vi "Initialize lock in.vi"(6 "Internal Reference Frequency (1000 Hz)":dbl=1000.0, 7 "Sine Output Amplitude (1 V)":dbl=1.0, 9 "Data Collection":T2={"Sample Rate (0: 62.5 mHz)"=0, "Continuous Storage (T: Enable)"=TRUE, "Number of Points (100)"=100, "Channel (1: Channel 1 Display)"=1, "Channel 1 Display (0: X)"=0} {"Channel 1 Display (0: X)" items=["X", "R", "X Noise", "Aux In 1", "Aux In 2"]; "Channel (1: Channel 1 Display)" items=["Channel 1 Display"=1, "Channel 2 Display"=2]; "Sample Rate (0: 62.5 mHz)" items=["62.5 mHz", "125 mHz", "250 mHz", "500 mHz", "1 Hz", "2 Hz", "4 Hz", "8Hz", "16 Hz", "32 Hz", "64 Hz", "128 Hz", "256 Hz", "512 Hz", "Trigger "]}, 11 "Configure":T3={"Lock in Amplifier PORT"="", "Input Connection (0: Single-Ended Voltage) "=0, "Input Coupling (0: AC)"=0, "Input Notch Filter (0: None)"=0, "Reference Source (1: Internal)"=1, "Dynamic Reserve (-1: Auto Reserve)"=-1, "Sensitivity (-1: Auto gain)"=-1, "Time Constant (8: 100ms)"=8} {"Time Constant (8: 100ms)" items=["10 us", "30 us", "100 us", "300 us", "1 ms", "3 ms", "10 ms", "30 ms", "100 ms", "300 ms", "1 s", "3 s", "10 s", "30 s", "100 s", "300 s", "1 ks", "3 ks", "10 ks", "30 ks"]; "Sensitivity (-1: Auto gain)" items=["Auto Gain"=-1, "2 nV/fA"=0, "5 nV/fA"=1, "10 nV/fA"=2, "20 nV/fA"=3, "50 nV/fA"=4, "100 nV/fA"=5, "200 nV/fA"=6, "500 nV/fA"=7, "1 uV/pA"=8, "2 uV/pA"=9, "5 uV/pA"=10, "10 uV/pA"=11, "20 uV/pA"=12, "50 uV/pA"=13, "100 uV/pA"=14, "200 uV/pA"=15, "500 uV/pA"=16, "1 mV/nA"=17, "2 mV/nA"=18, "5 mV/nA"=19, "10 mV/nA"=20, "20 mV/nA"=21, "50 mV/nA"=22, "100 mV/nA"=23, "200 mV/nA"=24, "500 mV/mA"=25, "1 V/uA"=26]; "Dynamic Reserve (-1: Auto Reserve)" items=["Auto Reserve"=-1, "High Reserve"=0, "Normal"=1, "Low Noise"=2]; "Reference Source (1: Internal)" items=["External", "Internal"]; "Input Notch Filter (0: None)" items=["None", "Line Notch", "2x Line Notch", "Both Notch Filters"]; "Input Coupling (0: AC)" items=["AC", "DC"]; "Input Connection (0: Single-Ended Voltage)" items=["Single-Ended Voltage", "Differential Voltage", "1 MOhm Current Gain", "100 MOhm Current Gain"]}) -> (1 "Output":T1)   [LabVIEW 2020]
uses:
  Downloads/stanford_research_830/Stanford Research 830/Stanford Research 830.lvlib
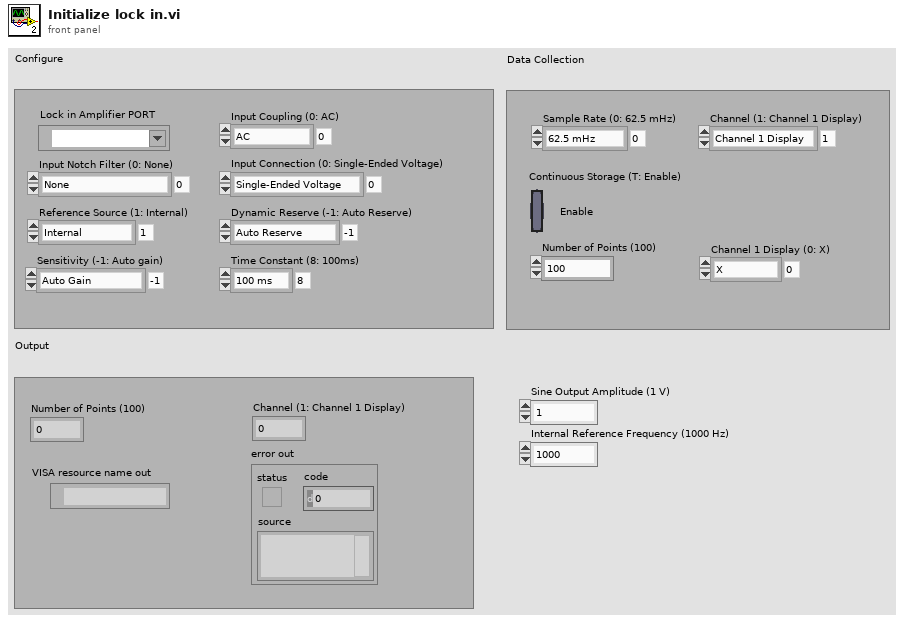
[diagram p1: front panel]
types:
  T1 = cluster{"Number of Points (100)":u32, "VISA resource name out":refnum<visa-resource-name>, "Channel (1: Channel 1 Display)":u16, "error out":errorcluster}
  T2 = cluster{"Sample Rate (0: 62.5 mHz)":u16, "Continuous Storage (T: Enable)":bool, "Number of Points (100)":u32, "Channel (1: Channel 1 Display)":u16, "Channel 1 Display (0: X)":u16}
  T3 = cluster{"Lock in Amplifier PORT":refnum<visa-resource-name>, "Input Connection (0: Single-Ended Voltage) ":u16, "Input Coupling (0: AC)":u16, "Input Notch Filter (0: None)":u16, "Reference Source (1: Internal)":u16, "Dynamic Reserve (-1: Auto Reserve)":i16, "Sensitivity (-1: Auto gain)":i16, "Time Constant (8: 100ms)":u16}
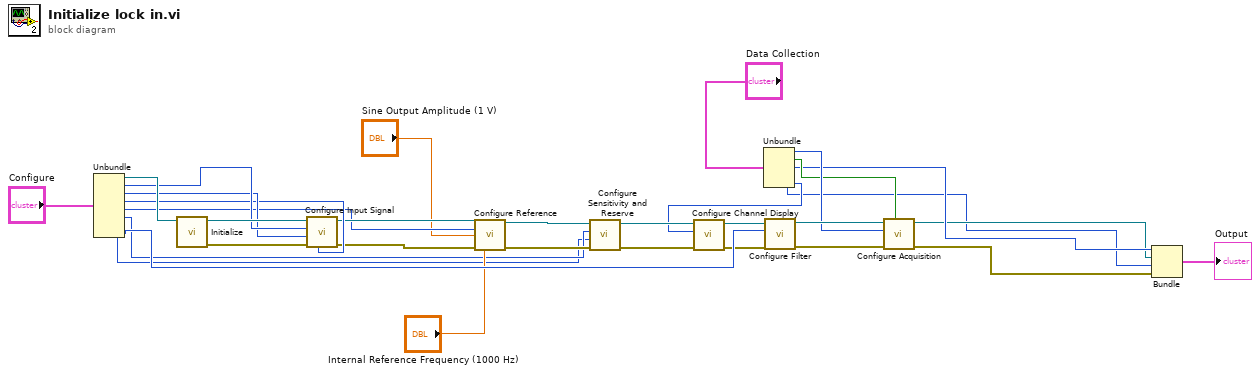
[diagram p0: block diagram]
diagram:
  n1 = Unbundle("Configure") -> ("Lock in Amplifier PORT"=w29:refnum<visa-resource-name>, "Input Connection (0: Single-Ended Voltage)"=w28:u16, "Input Coupling (0: AC)"=w27:u16, "Input Notch Filter (0: None)"=w26:u16, "Reference Source (1: Internal)"=w20:u16, "Dynamic Reserve (-1: Auto Reserve)"=w12:i16, "Sensitivity (-1: Auto gain)"=w11:i16, "Time Constant (8: 100ms)"=w18:u16)
  n2 = call "Initialize.vi"("VISA resource name"=w29) -> ("error out"=w31:errorcluster, "VISA resource name out"=w32:refnum<visa-resource-name>)  [unwired: 9 in]
  n3 = call "Configure Input Signal.vi"("Input Notch Filter (0: None)"=w26, "error in (no error)"=w31, "Input Coupling (0: AC)"=w27, "Input Connection (0: Single-Ended Voltage)"=w28, "VISA resource name"=w32) -> ("error out"=w19:errorcluster, "VISA resource name out"=w23:refnum<visa-resource-name>)  [unwired: 5 in]
  n4 = call "Configure Reference.vi"("VISA resource name"=w23, "Reference Source (1: Internal)"=w20, "Sine Output Amplitude (1 V)"="Sine Output Amplitude (1 V)", "error in (no error)"=w19, "Internal Reference Frequency (1000 Hz)"="Internal Reference Frequency (1000 Hz)") -> ("VISA resource name out"=w22:refnum<visa-resource-name>, "error out"=w21:errorcluster)  [unwired: 9 in]
  n5 = call "Configure Sensitivity and Reserve.vi"("error in (no error)"=w21, "Sensitivity (-1: Auto gain)"=w11, "Dynamic Reserve (-1: Auto Reserve)"=w12, "VISA resource name"=w22) -> ("error out"=w7:errorcluster, "VISA resource name out"=w8:refnum<visa-resource-name>)  [unwired: 6 in]
  n6 = Unbundle("Data Collection") -> ("Sample Rate (0: 62.5 mHz)"=w16:u16, "Continuous Storage (T: Enable)"=w15:bool, "Number of Points (100)"=w3:u32, "Channel (1: Channel 1 Display)"=w1:u16, "Channel 1 Display (0: X)"=w6:u16)
  n7 = call "Configure Channel Display.vi"("error in (no error)"=w7, "Channel 1 Display (0: X)"=w6, "VISA resource name"=w8) -> ("error out"=w9:errorcluster, "VISA resource name out"=w10:refnum<visa-resource-name>)  [unwired: 7 in]
  n8 = call "Configure Filter.vi"("error in (no error)"=w9, "Time Constant (8: 100ms)"=w18, "VISA resource name"=w10) -> ("error out"=w24:errorcluster, "VISA resource name out"=w25:refnum<visa-resource-name>)  [unwired: 7 in]
  n9 = call "Configure Acquisition.vi"("Continuous Storage (T: Enable)"=w15, "error in (no error)"=w24, "Sample Rate (0: 62.5 mHz)"=w16, "VISA resource name"=w25) -> ("error out"=w4:errorcluster, "VISA resource name out"=w2:refnum<visa-resource-name>)  [unwired: 6 in]
  n10 = Bundle("Number of Points (100)"=w3, "VISA resource name out"=w2, "Channel (1: Channel 1 Display)"=w1, "error out"=w4) -> (→"Output":T1)  [unwired: 1 in]
